vi "VISA Send Query.vi"(8 "error in":errorcluster, 10 "Query":string, 11 "34980A in":refnum<class "34980A.lvclass">) -> (0 "error out":errorcluster, 2 "read buffer":string, 3 "34980A out":refnum<class "34980A.lvclass">)   [LabVIEW 2019, in "34980A.lvlib" / "34980A.lvclass"]
uses:
  Library/34980A.lvclass
  Library/34980A.lvclass/34980A.ctl
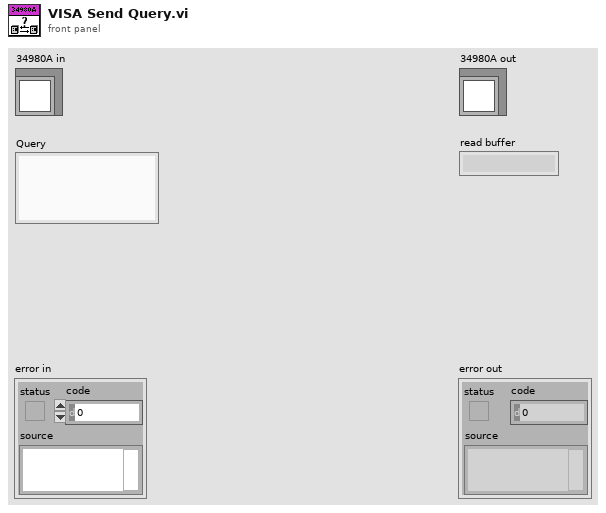
[diagram p1: front panel]
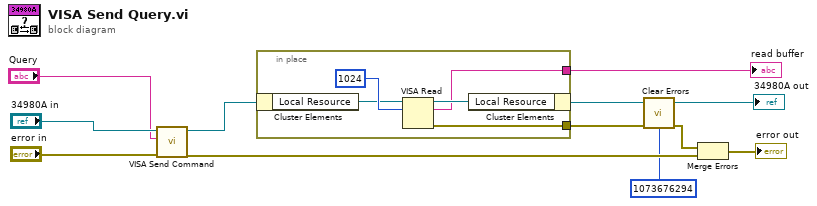
[diagram p0: block diagram]
diagram:
  n1 = call "VISA Send Command.vi"("error in"="error in", "Command"="Query", "34980A in"="34980A in") -> ("error out"=w6:errorcluster, "34980A out"=w8:refnum<class "34980A.lvclass">)  [unwired: 7 in]
  n2 = in-place {
    in-place-border: [w14] -> w2
    in-place-border: [w13] -> w4
    n3 = in-place-cluster #1(w8) -> ("Local Resource"=w12:refnum<visa-resource-name>)
    n4 = VISA Read(VISA resource name=w12, byte count=u32 1024) -> (VISA resource name out=w16:refnum<visa-resource-name>, read buffer=w13:string, error out=w14:errorcluster)  [unwired: 1 in, 1 out]
    n5 = in-place-cluster #1("Local Resource"=w16) -> (→"34980A out":refnum<class "34980A.lvclass">)
  }
  "read buffer" <- w4
  n6 = call <vilib>:"Clear Errors.vi"("error in (no error)"=w2, "specific error code to clear (0: all)"=1073676294) -> ("error out"=w1:errorcluster)  [unwired: 4 in, 1 out]
  n7 = Merge Errors(w1, w6) -> (→"error out":errorcluster)
